vi "Destroy Server.vi"(8 "error in (no error)":errorcluster, 11 "gRPC Server in":refnum<class "gRPC Server.lvclass">) -> (0 "error out":errorcluster, 3 "gRPC Server out":refnum<class "gRPC Server.lvclass">)   [LabVIEW 2019, in "gRPC Server (scope.proto).lvlib" / "gRPC Server.lvclass"]
uses:
  gRPC Server.lvclass
  <vilib>/gRPC/LabVIEW gRPC Servicer/Servicer/Servicer.lvclass
  <vilib>/gRPC/LabVIEW gRPC Library/grpc-lvsupport-release.lvlib
  <vilib>/gRPC/LabVIEW gRPC Servicer/ServiceBase/ServiceBase.lvclass
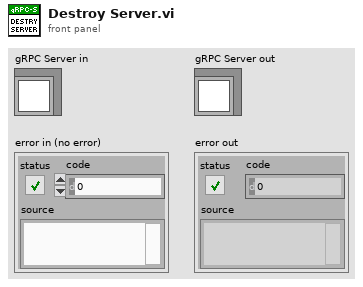
[diagram p1: front panel]
types:
  T1 = typedef "grpc-lvsupport-release.lvlib/grpcId.ctl" = u64
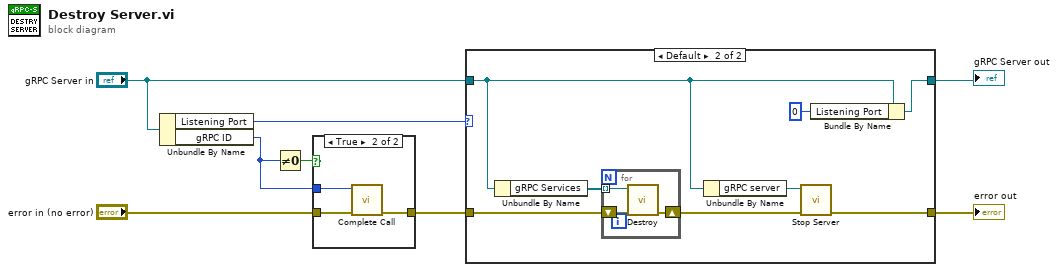
[diagram p0: block diagram]
diagram:
  n1 = Unbundle By Name("gRPC Server in") -> ("Listening Port"=w8:i32, "gRPC ID"=w1:T1)
  n2 = Not Equal To 0?(x=w1) -> (x != 0?=w2:bool)
  n3 = case shown="True" w2 {
    tunnel: "error in (no error)" -> [w9 w12]
    tunnel: [w9 w11] -> w3
    tunnel: w1 -> [_ w10]
    frame False {
    }
    frame True {
      n4 = call <vilib>:"Complete Call.vi"("gRPCid"=w10, "error in"=w12) -> ("error out"=w11:errorcluster)  [unwired: 8 in]
    }
  }
  n5 = case shown="Default" w8 {
    tunnel: w3 -> [w14 w18]
    tunnel: [w14 w21] -> w6
    tunnel: "gRPC Server in" -> [w13 w16]
    tunnel: [w13 w19] -> w5
    frame 0 {
    }
    frame Default {
      n6 = Unbundle By Name(w16) -> ("gRPC Services"=w15:refnum<class "ServiceBase.lvclass">[])
      n7 = for {
        tunnel: w15 -> [w23] mode=indexing
        shift-right: [w24] -> w17
        shift-left: w18 -> [w25]
        n8 = call-dynamic "Destroy.vi"("error in"=w25, "gRPC service in"=w23) -> ("error out"=w24:errorcluster)  [unwired: 8 in, 1 out]
      }
      n9 = Unbundle By Name(w16) -> ("gRPC server"=w22:refnum<class "Servicer.lvclass">)
      n10 = call <vilib>:"Stop Server.vi"("error in"=w17, "gRPC server in"=w22) -> ("error out"=w21:errorcluster)  [unwired: 9 in]
      n11 = Bundle By Name(cluster=w16, "Listening Port"=0) -> (w19:refnum<class "gRPC Server.lvclass">)
    }
  }
  "error out" <- w6
  "gRPC Server out" <- w5
